vi "Random Burn.vi"(11 "Pixel Array In":i32[](array[numeric])) -> (3 "Pixel Array Out":i32[](array[numeric]))   [LabVIEW 2019]
doc: "Removes the fire image source by randomly decreasing its intensity until it is removed completely. Repeated calls to Do Fire.vi will then burn up the remainder of the fire."
uses:
  <vilib>/numeric/Random Number (Range) U64.vi
  <vilib>/numeric/sub_Random U32.vi
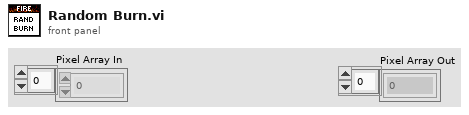
[diagram p1: front panel]
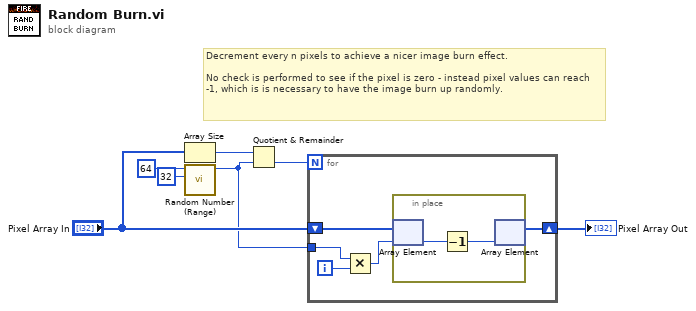
[diagram p0: block diagram]
diagram:
  # "Decrement every n pixels to achieve a nicer image burn effect.\n\nNo check is performed to see if the pixel is zero - instead pixel values can reach -1, which is is necessary to have the image burn up randomly."
  n1 = Array Size(array="Pixel Array In") -> (size(s)=w3:i32)
  n2 = call-poly <vilib>:"Random Number (Range).vi"("lower bound (0)"=u64 32, "upper bound (100)"=u64 64) -> ("number"=w1:u64)  [unwired: 9 in]
  n3 = Quotient & Remainder(x=w3, y=w1) -> (floor(x/y)=w2:u64)  [unwired: 1 out]
  n4 = for {
    N: w2 -> [_]
    shift-right: [w8] -> w7
    shift-left: "Pixel Array In" -> [w12]
    tunnel: w1 -> [w10]
    i -> [w11]
    n5 = Multiply(x=w10, y=w11) -> (x*y=w9:u64)
    n6 = in-place {
      n7 = in-place-array #1(w12, w9) -> (w14:i32)
      n8 = Decrement(x=w14) -> (x-1=w13:i32)
      n9 = in-place-array #1(w13) -> (w8:i32[])  [unwired: 1 out]
    }
  }
  "Pixel Array Out" <- w7
